vi "Sub Super Duper_14_02_18_JWa.vi"(0 "VISA resource name":refnum<visa-resource-name>="GPIB0::17::INSTR", 1 "Sample Properties:":T9 {"Date Created" format="%<%Y/%m/%d>T"}, 2 "Gated SMU4 is...":bool, 3 "TRF Cluster":T10={"Step 4"=-38.0, "# of Loops"=1.0, "Transfer 2"=FALSE, "Start 4"=-2.0, "Total Points 2"=2, "Start 3"=40.0, "Stop 2"=-40.0, "Step 3"=-1.0, "Loop Step"=0.0, "Integration Time 3"=0, "Loop Wait"=0.0, "First Step"=0.0} {"Loop Wait" format="%<%H:%M:%S>t"; "Integration Time 3" scale=0.0..2.0; "Step 3" format="%.2f"; "Stop 2" format="%.2f"; "Start 3" format="%.2f"; "Start 4" format="%.2f"; "Step 4" format="%.2f"}, 4 "TSP Cluster":T11={"Transport"=FALSE, "Start 2"=0.0, "Stop 3"=-60.0, "Step 2"=-1.0, "Start"=0.0, "Step"=-10.0, "Total Points"=7, "Integration Time"=0} {"Integration Time" scale=0.0..2.0; "Step" format="%.2f"; "Start" format="%.2f"; "Step 2" format="%.2f"; "Stop 3" format="%.2f"; "Start 2" format="%.2f"}, 5 "Compliance Cluster":T6={"Var1 sweep settings"={"sweep spacing (linear: 0)"=0, "sweep mode"=FALSE, "compliance (V)"=100.0, "compliance (A)"=0.001}, "Var1 sweep settings 2"={"sweep spacing (linear: 0)"=0, "sweep mode"=FALSE, "compliance (V)"=100.0, "compliance (A)"=0.001}, "Var2 step settings 2"={"compliance (A)"=0.001, "compliance (V)"=100.0}, "Var2 step settings"={"compliance (A)"=0.001, "compliance (V)"=100.0}} {"Var2 step settings"."compliance (V)" format="%.2f"; "Var2 step settings"."compliance (A)" format="%^.2e"; "Var2 step settings 2"."compliance (V)" format="%.2f"; "Var2 step settings 2"."compliance (A)" format="%^.2e"; "Var1 sweep settings 2"."compliance (A)" format="%^.2e"; "Var1 sweep settings 2"."compliance (V)" format="%.2f"; "Var1 sweep settings 2"."sweep spacing (linear: 0)" items=["linear", "log 10", "log 25", "log 50"]; "Var1 sweep settings"."compliance (A)" format="%^.2e"; "Var1 sweep settings"."compliance (V)" format="%.2f"; "Var1 sweep settings"."sweep spacing (linear: 0)" items=["linear", "log 10", "log 25", "log 50"]}, 6 "Light Bathe Cluster":T2={"TG to BG:  "=FALSE, "TG to BG Durration"=120.0, "TRF to TSP:   "=FALSE, "TRF to TSP Duration"=120.0, "Post Measure: "=FALSE, "TG to BG (TSP):"=FALSE, "TG to BG Durration 3"=120.0} {"TG to BG Durration 3" format="%<%H:%M:%S>t"; "TRF to TSP Duration" format="%<%H:%M:%S>t"; "TG to BG Durration" format="%<%H:%M:%S>t"}, 7 "error in":errorcluster, 8 "Saved Folder:":path=path "C:/1DATA/2011", 9 "Wait Cluster":T5 {"Wait Time (s)" format="%.1g"; "Wait Countdown" format="%<%H:%M:%S%1u>t"}, 11 "TG Dielectric Prop":T1, 13 "Stop \nCountdown":bool, 15 "Loop Count":dbl, 16 "Gate Current Cluster":T3={"Gate Current (TSP)"={"Y2 axis on/off"=FALSE, "MINIMUM"=0.0, "MAXIMUM"=1.0, "Variable name"="Ig", "LIN or LOG axis"="LIN"}, "Gate Current (TRF)"={"Y2 axis on/off"=FALSE, "MINIMUM"=0.0, "MAXIMUM"=1.0, "Variable name"="Ig", "LIN or LOG axis"="LIN"}} {"Gate Current (TSP)"."MAXIMUM" format="%.9f"; "Gate Current (TSP)"."MINIMUM" format="%.9f"; "Gate Current (TRF)"."MAXIMUM" format="%.9f"; "Gate Current (TRF)"."MINIMUM" format="%.9f"}, 17 "Dielectric Constant (BG)":dbl) -> (12 "Status Indicator":bool, 14 "Vt Cluster":T4 {"Id Max" format="%.3g"; "Vt Max" format="%.3g"; "Vt Min" format="%.3g"; "Vt Ratio" format="%.3g"}, 20 "VISA resource name out":refnum<visa-resource-name>, 21 "TRF Path":path, 23 "TSP Path":path, 24 "Graph Cluster":T7, 25 "Char Cluster":T8 {"Mobility-Lin" format="%#_4e"; "On/Off" format="%#_4e"; "Mobility-Sat" format="%#_4e"}, 27 "error out":errorcluster)   [LabVIEW 2012]
uses:
  <vilib>/Platform/TimedLoop/XDataNode/wakeup.ctl
  <vilib>/Platform/TimedLoop/XDataNode/XDNodeRunTimeDep.lvlib
  <vilib>/Platform/TimedLoop/XDataNode/nitl_modes.ctl
  <vilib>/Platform/TimedLoop/XDataNode/timing_clust.ctl
  <vilib>/Platform/TimedLoop/XDataNode/XDataNode.xnode
panel:
  out "LKG Path":path
  # "Vg Sweep"
  # "Vd Step"
  # "Loops and Integration Time"
  # "Device Characteristics"
  # "Light Bath is..."
  # "Duration (hh:mm:ss)"
  # "Sample Properties:"
  # "%"
  # "nm"
  # "Device Properties:"
  # "um"
  # "um"
  # "Vg Step"
  # "Vd Step"
  # "Integration Time"
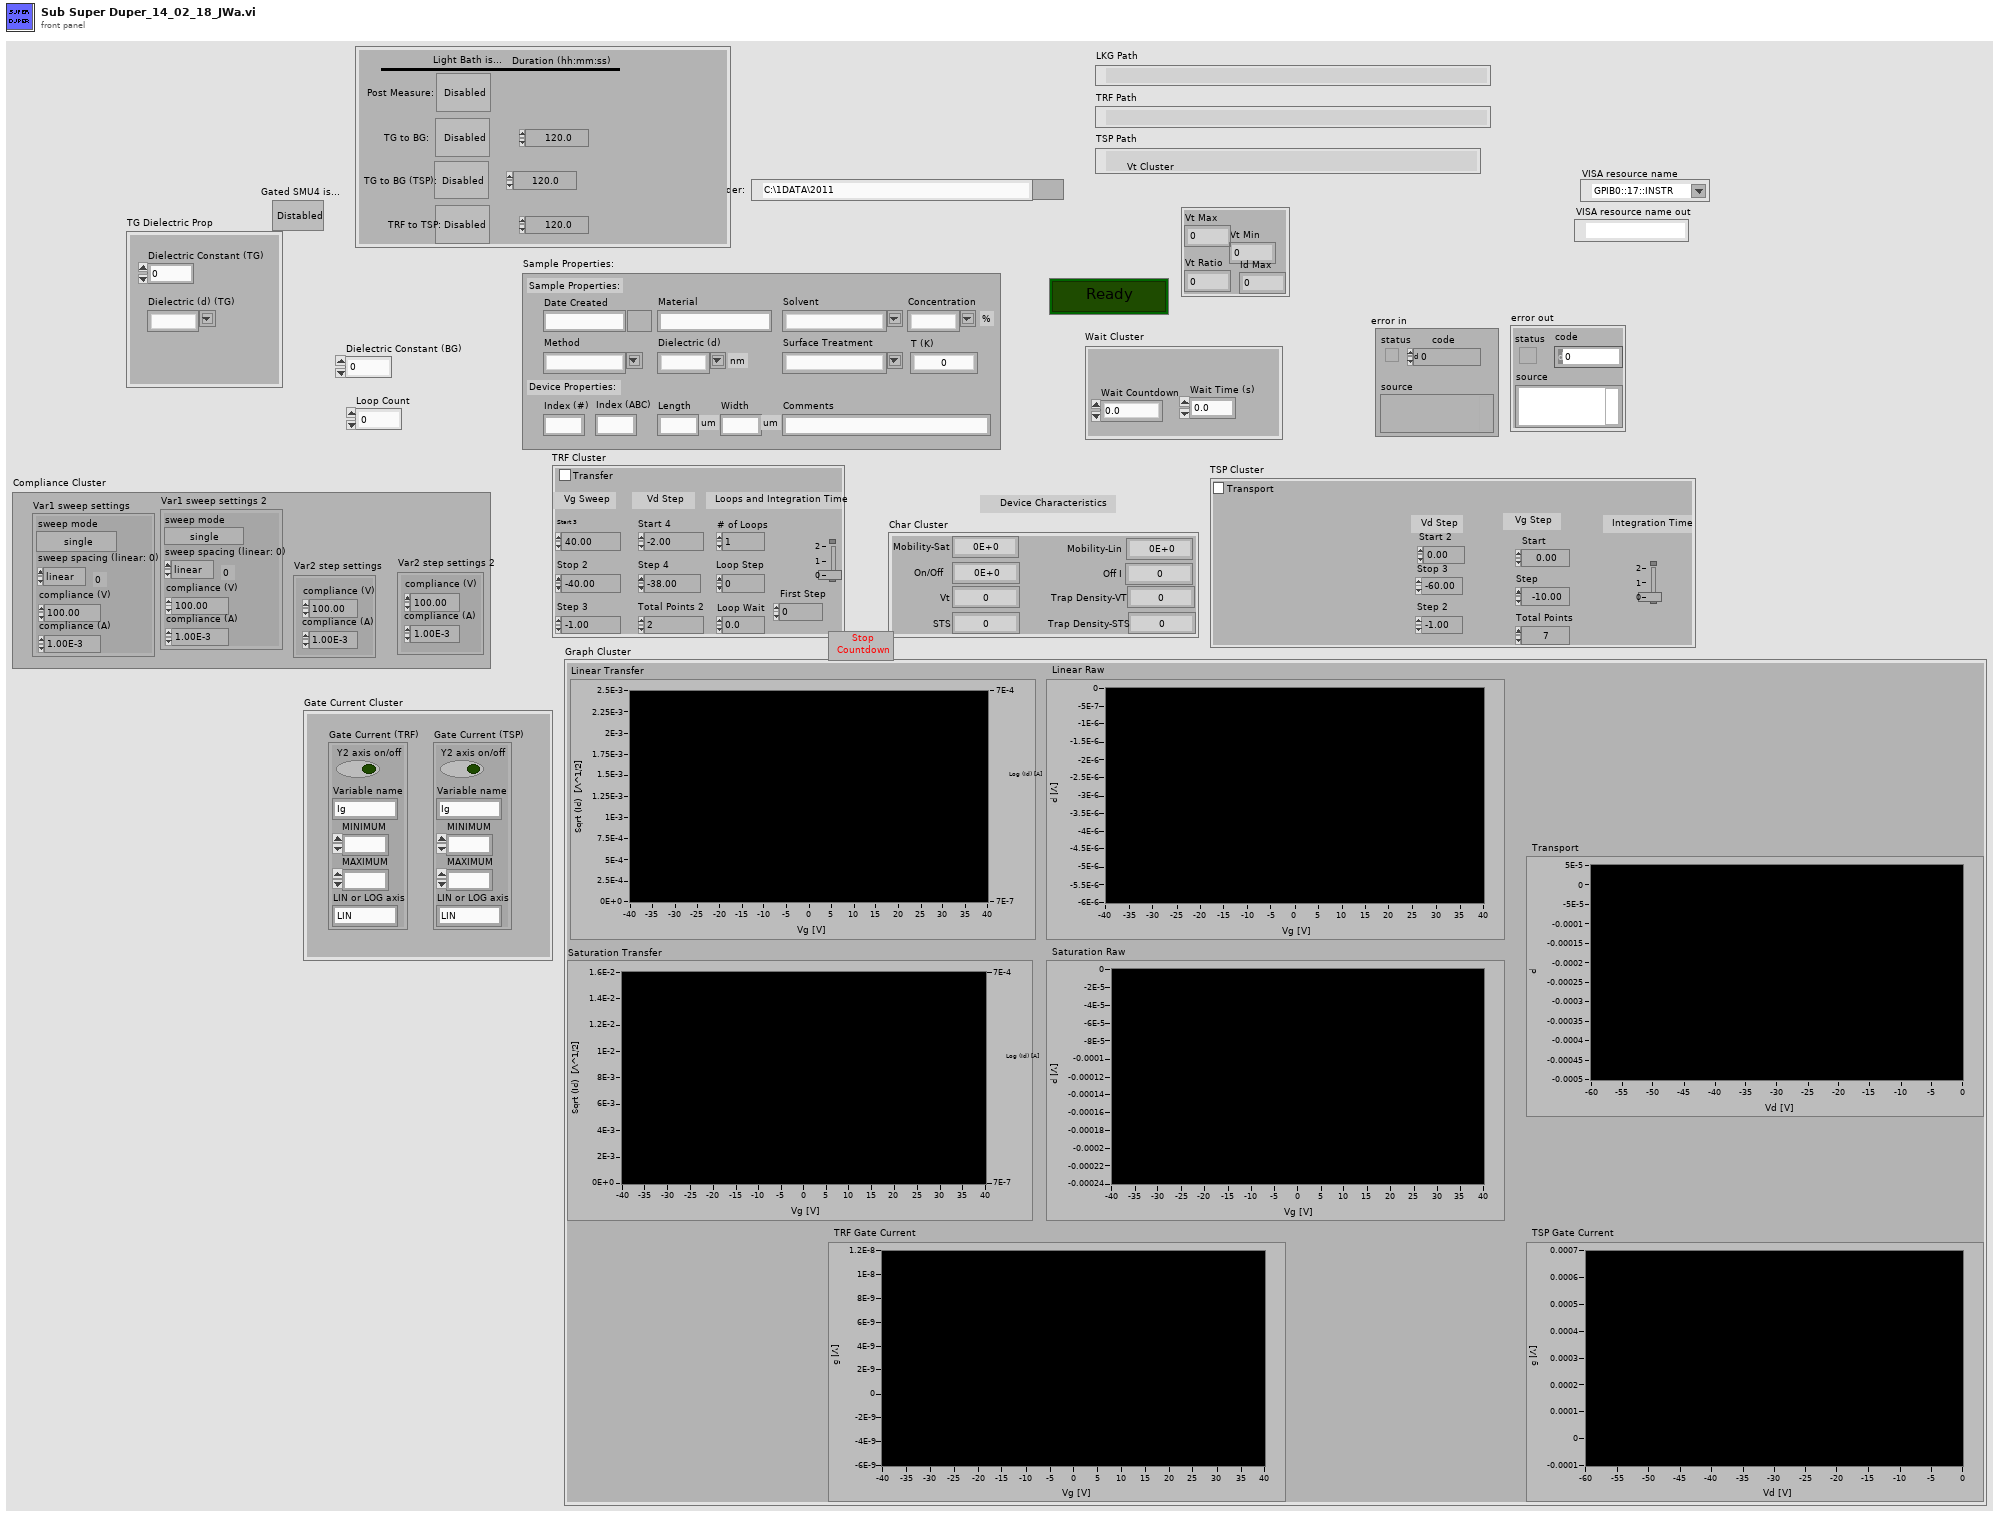
[diagram p1: front panel]
types:
  T1 = cluster{"Dielectric Constant (TG)":dbl, "Dielectric (d) (TG)":string}
  T2 = cluster{"TG to BG:  ":bool, "TG to BG Durration":dbl, "TRF to TSP:   ":bool, "TRF to TSP Duration":dbl, "Post Measure: ":bool, "TG to BG (TSP):":bool, "TG to BG Durration 3":dbl}
  T3 = cluster{"Gate Current (TSP)":cluster{"Y2 axis on/off":bool, "MINIMUM":ext, "MAXIMUM":ext, "Variable name":string, "LIN or LOG axis":string}, "Gate Current (TRF)":cluster{"Y2 axis on/off":bool, "MINIMUM":ext, "MAXIMUM":ext, "Variable name":string, "LIN or LOG axis":string}}
  T4 = cluster{"Vt Max":i32, "Vt Min":i32, "Vt Ratio":i32, "Id Max":i32}
  T5 = cluster{"Wait Countdown":dbl, "Wait Time (s)":dbl}
  T6 = cluster{"Var1 sweep settings":cluster{"sweep spacing (linear: 0)":u16, "sweep mode":bool, "compliance (V)":dbl, "compliance (A)":dbl}, "Var1 sweep settings 2":cluster{"sweep spacing (linear: 0)":u16, "sweep mode":bool, "compliance (V)":dbl, "compliance (A)":dbl}, "Var2 step settings 2":cluster{"compliance (A)":dbl, "compliance (V)":dbl}, "Var2 step settings":cluster{"compliance (A)":dbl, "compliance (V)":dbl}}
  T7 = cluster{"Linear Transfer":cluster{dbl[], "trace":dbl[]}[], "Linear Raw":cluster{dbl[], dbl[]}[], "Saturation Transfer":cluster{dbl[], "trace":dbl[]}[], "Saturation Raw":cluster{dbl[], dbl[]}[], "Transport":cluster{dbl[], dbl[]}[], "TRF Gate Current":cluster{dbl[], dbl[]}[], "TSP Gate Current":cluster{dbl[], dbl[]}[]}
  T8 = cluster{"Mobility-Sat":dbl, "Mobility-Lin":dbl, "On/Off ":dbl, "Off I":dbl, "Vt":dbl, "STS":dbl, "Trap Density-VT":dbl, "Trap Density-STS":dbl}
  T9 = cluster{"Date Created":timestamp, "Material":string, "Solvent":string, "Concentration":string, "Method":string, "Dielectric (d)":string, "Index (#)":string, "Index (ABC)":string, "Length":string, "Width":string, "Surface Treatment":string, "Comments":string, "T (K)":dbl}
  T10 = cluster{"Step 4":dbl, "# of Loops":dbl, "Transfer 2":bool, "Start 4":dbl, "Total Points 2":u16, "Start 3":dbl, "Stop 2":dbl, "Step 3":dbl, "Loop Step":dbl, "Integration Time 3":u32, "Loop Wait":dbl, "First Step":dbl}
  T11 = cluster{"Transport":bool, "Start 2":dbl, "Stop 3":dbl, "Step 2":dbl, "Start":dbl, "Step":dbl, "Total Points":u16, "Integration Time":u32}
  T12 = typedef "XDNodeRunTimeDep.lvlib/timing_clust.ctl" = cluster{"Expected End [f-1]":u64, "Actual End [f-1]":u64, "Finished Late? [f-1]":bool, "Expected End [i-1]":u64, "Actual End [i-1]":u64, "Finished Late? [i-1]":bool, "Expected Start [i]":u64, "Actual Start [i]":u64, "Expected Start [f]":u64, "Actual Start [f]":u64, "Source Name":string, "Structure Name":string, "Period":i64, "Deadline":i64, "Offset":i64, "Start":i64, "Priority":i32, "Timeout":i32, "Mode":T13, "Wakeup Reason":T14, "Error":errorcluster, "Source Type":string, "Secondary Source Type":string, "Global End Time":u64, "Global Start Time":u64, "Frame Duration":u64, "Iteration Duration":u64, "Assigned CPU":i32, "I/O Scan Engine Mode":u32}
  T13 = typedef "XDNodeRunTimeDep.lvlib/nitl_modes.ctl" = enum32{"No Change", "Process missed periods, maintain original phase", "Discard missed periods, maintain original phase", "Process missed periods, ignore original phase", "Discard missed periods, ignore original phase"}
  T14 = typedef "XDNodeRunTimeDep.lvlib/wakeup.ctl" = enum32{"Normal", "Aborted", "Asynchronous wakeup", "Timing source error", "Timed loop error", "Timeout"}
  T15 = cluster{"sweep spacing (linear: 0)":u16, "sweep mode":bool, "compliance (V)":dbl, "compliance (A)":dbl}
  T16 = cluster{"compliance (A)":dbl, "compliance (V)":dbl}
  T17 = cluster{"Y2 axis on/off":bool, "MINIMUM":ext, "MAXIMUM":ext, "Variable name":string, "LIN or LOG axis":string}
  T18 = cluster{"Start 3":dbl, "Stop 2":dbl, "Step 3":dbl, "sweep spacing (linear: 0)":u16, "sweep mode":bool, "compliance (V)":dbl, "compliance (A)":dbl}
  T19 = cluster{"compliance (A)":dbl, "compliance (V)":dbl, "Start 4":dbl, "Total Points 2":u16, dbl}
  T20 = cluster{"Vt Max":i32, "Vt Min":i32, "Vt Ratio":i32, "Id Max":dbl}
  T21 = cluster{"Mobility-Sat":dbl, "Mobility-Lin":dbl, "On/Off Current":dbl, "Off I":dbl, "Vt":dbl, "STS":dbl, "Trap Density-VT":dbl, "Trap Density-STS":dbl}
  T22 = cluster{"Linear Sqrt":cluster{dbl[], "trace":dbl[]}[], "Linear Log":cluster{dbl[], "trace":dbl[]}[], "Linear Raw":cluster{dbl[], dbl[]}[], "Saturation Sqrt":cluster{dbl[], "trace":dbl[]}[], "Saturation Log":cluster{dbl[], "trace":dbl[]}[], "Saturation Raw":cluster{dbl[], "trace":dbl[]}[], "Gate Current":cluster{dbl[], "trace":dbl[]}[]}
  T23 = cluster{"Start 2":dbl, "Stop 3":dbl, "Step 2":dbl, "sweep spacing (linear: 0)":u16, "sweep mode":bool, "compliance (V)":dbl, "compliance (A)":dbl}
  T24 = cluster{"compliance (A)":dbl, "compliance (V)":dbl, "Start":dbl, "Total Points":u16, "Step":dbl}
  T25 = cluster{"Transport":cluster{dbl[], dbl[]}[], "Gate Current":cluster{dbl[], dbl[]}[]}
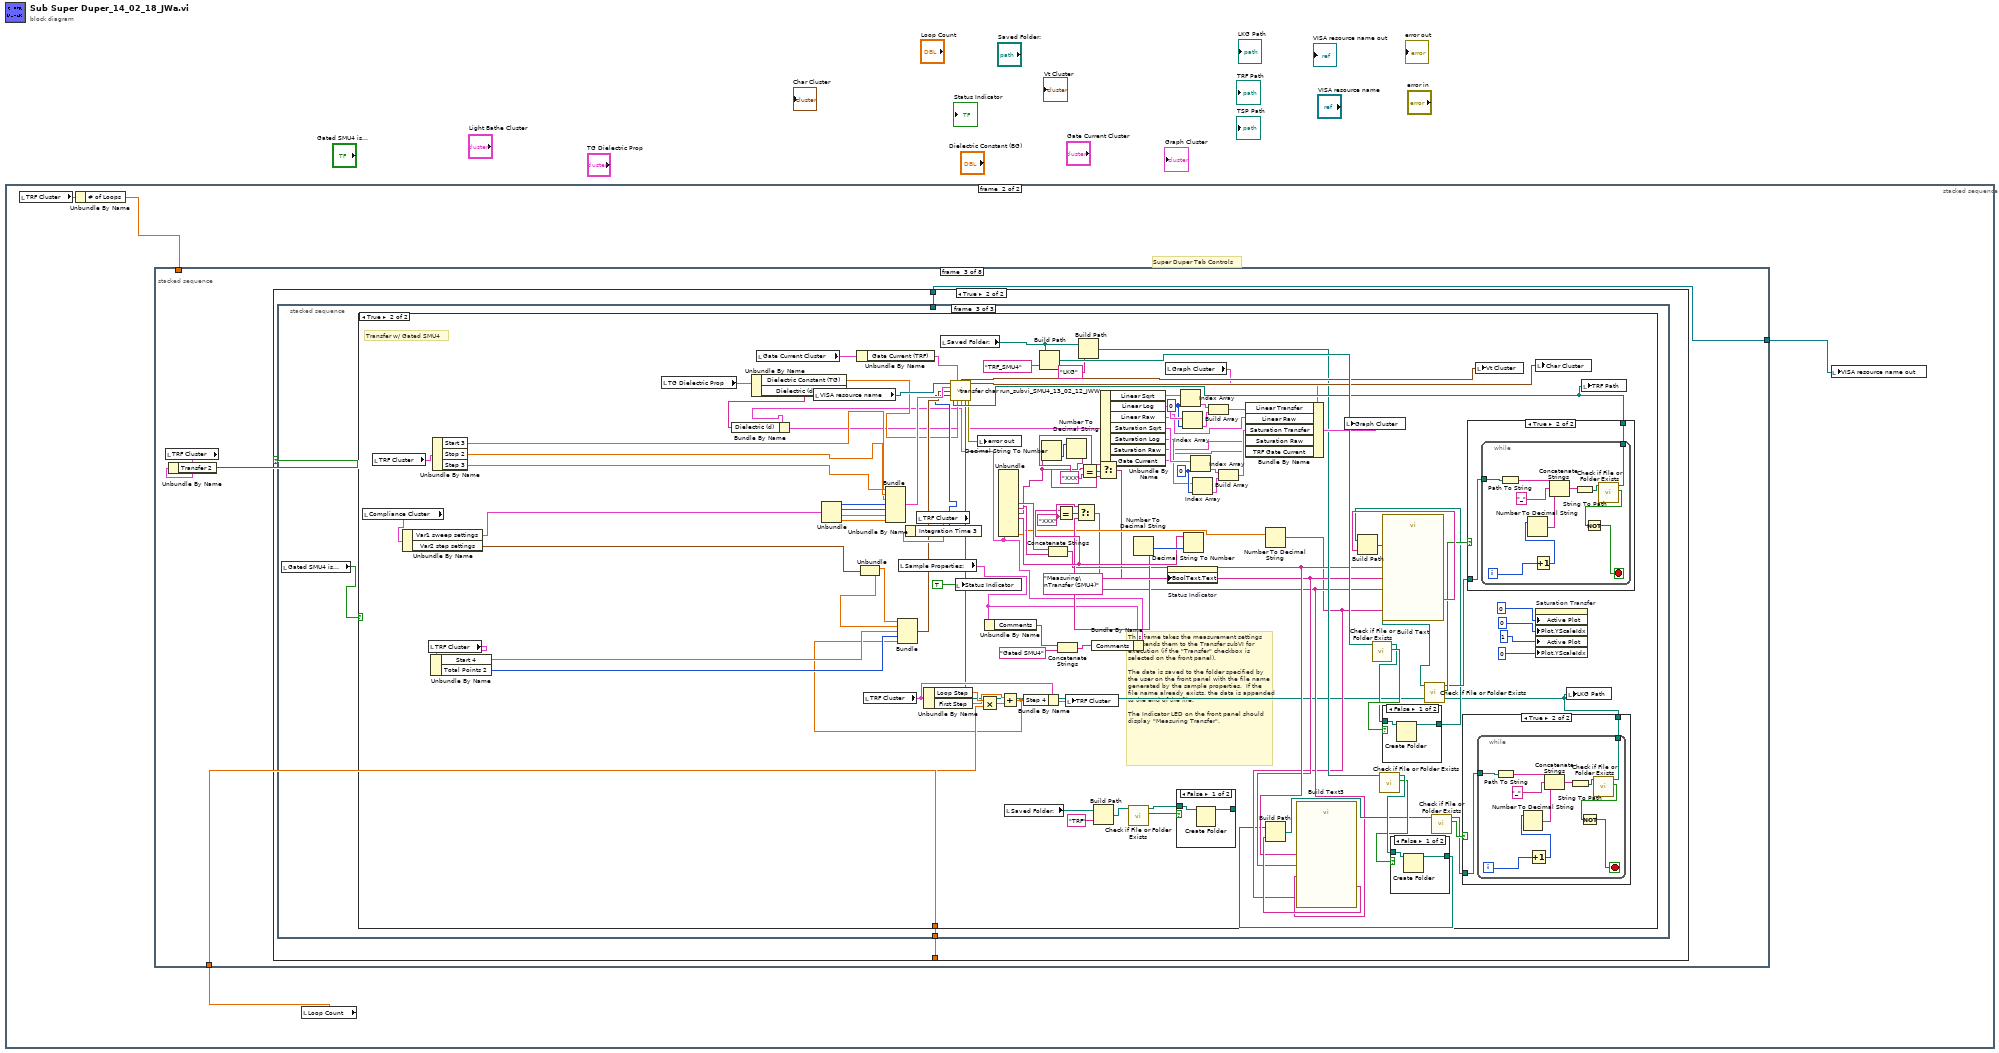
[diagram p0: block diagram]
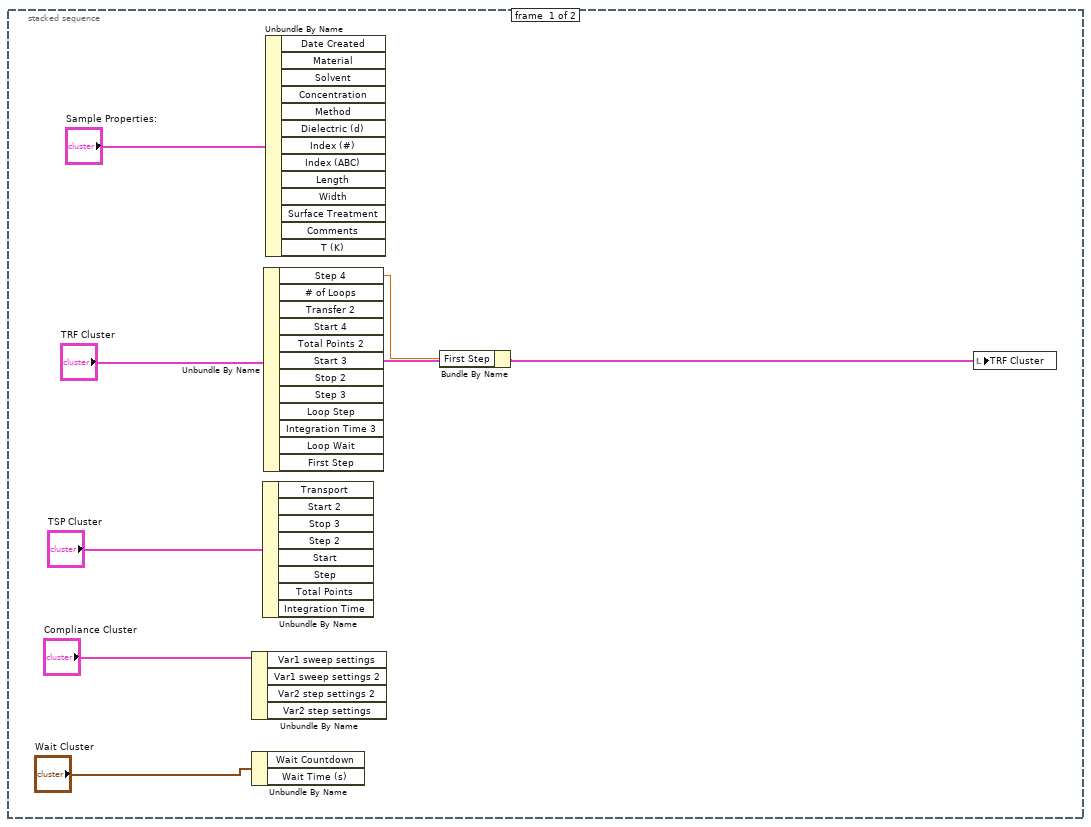
[diagram p2: hidden frame]
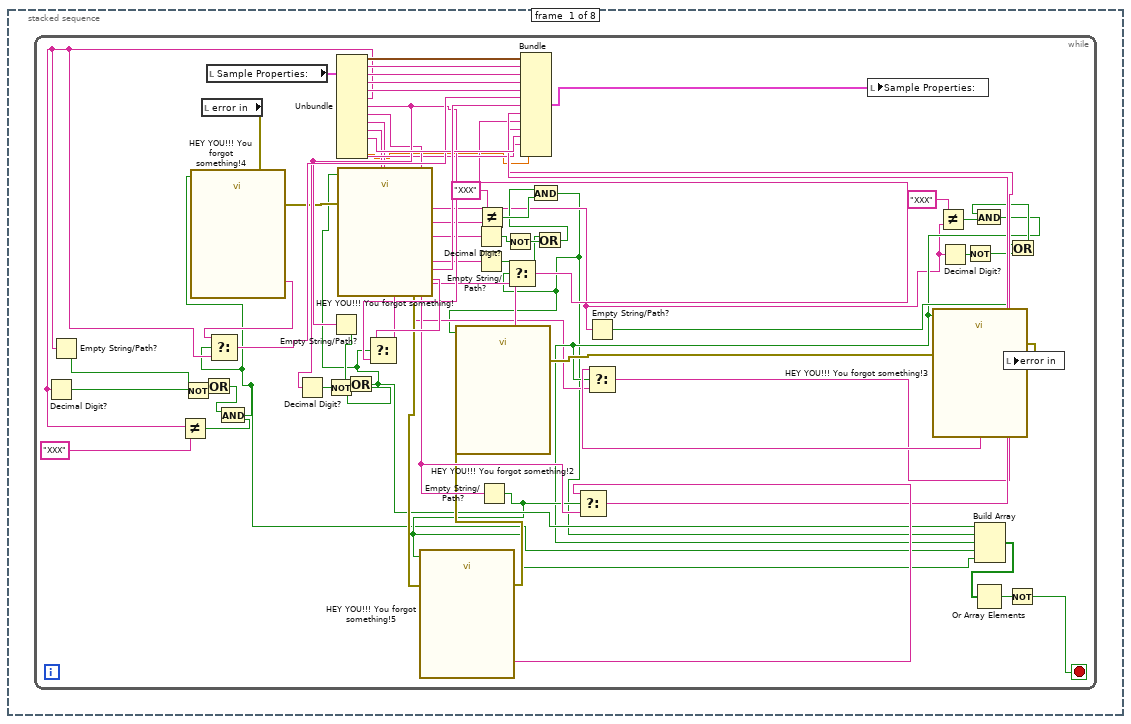
[diagram p3: hidden frame]
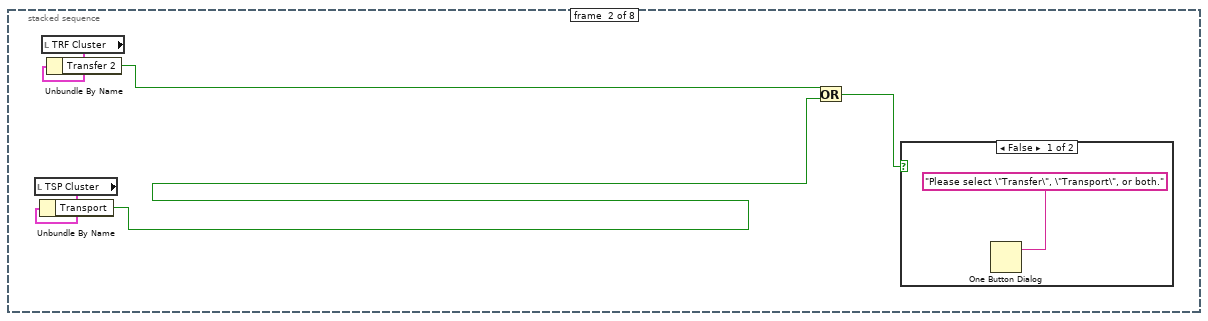
[diagram p4: hidden frame]
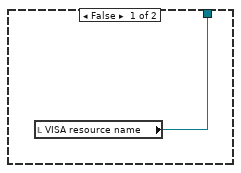
[diagram p6: hidden frame]
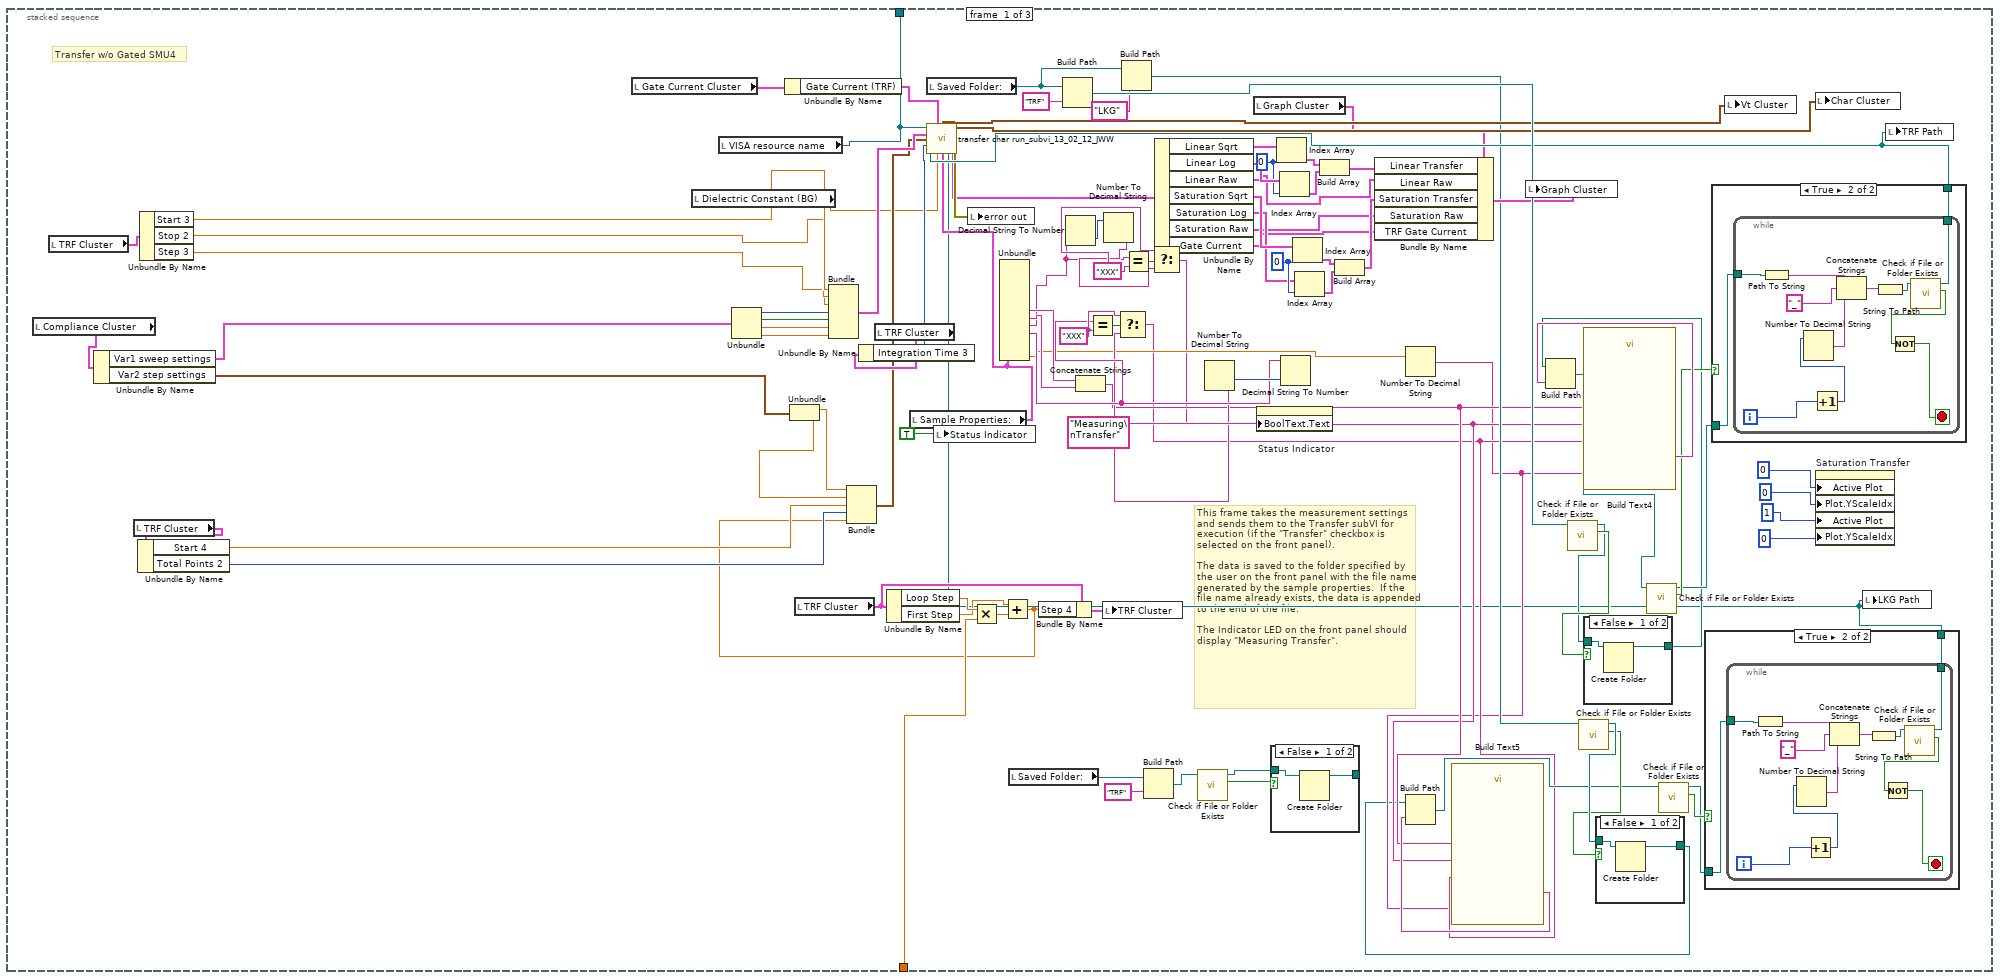
[diagram p7: hidden frame]
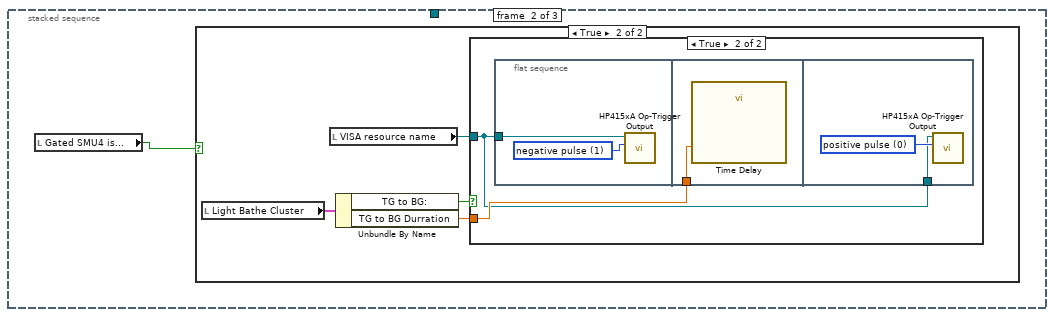
[diagram p13: hidden frame]
diagram:
  n1 = stacked-sequence {
    frame #0 {
      n2 = Unbundle By Name("Compliance Cluster") -> ()  [unwired: 4 out]
      n3 = Unbundle By Name("Wait Cluster") -> ()  [unwired: 2 out]
      n4 = Unbundle By Name("TSP Cluster") -> ()  [unwired: 8 out]
      n5 = Unbundle By Name("TRF Cluster") -> ("Step 4"=w7:dbl)  [unwired: 11 out]
      n6 = Unbundle By Name("Sample Properties:") -> ()  [unwired: 13 out]
      n7 = Bundle By Name(cluster="TRF Cluster", "First Step"=w7) -> (w5:T10)
      n8 = local write "TRF Cluster"(w5) -> ()
    }
    frame #1 {
      # "Super Duper Tab Controls"
      n9 = local read "TRF Cluster"() -> (w11:T10)
      n10 = Unbundle By Name(w11) -> ("# of Loops"=w10:dbl)
      n11 = local read "Loop Count"() -> (w8:dbl)
      n12 = stacked-sequence {
        tunnel: w8 -> [_ _ w81 _ _ _ _ w596]
        tunnel: w10 -> [_ _ _ _ _ _ _ w595]
        tunnel: [_ _ w78 _ _ _ _ _] -> w9
        frame #0 {
          n13 = while {
            stop <- w37 stop-if-true
            n14 = local read "error in"() -> (w43:errorcluster)
            n15 = local read "Sample Properties:"() -> (w66:T9)
            n16 = Unbundle(w66) -> ("Date Created"=w67:timestamp, "Material"=w68:string, "Solvent"=w69:string, "Concentration"=w70:string, "Method"=w71:string, "Dielectric (d)"=w26:string, "Index (#)"=w56:string, "Index (ABC)"=w53:string, "Length"=w21:string, "Width"=w14:string, "Surface Treatment"=w59:string, "Comments"=w51:string, "T (K)"=w12:dbl)
            n17 = Decimal Digit?(1:w26) -> (0:w34:bool)
            n18 = Empty String/Path?(string/path=w26) -> (empty?=w28:bool)
            n19 = Not Equal?(x=w26, y="XXX") -> (x != y?=w25:bool)
            n20 = Not(x=w34) -> (.not. x?=w31:bool)
            n21 = Or(x=w28, y=w31) -> (x .or. y?=w24:bool)
            n22 = And(x=w24, y=w25) -> (x .and. y?=w23:bool)
            n23 = call "HEY YOU!!! You forgot something!4"("Enable"=w23, "error in (no error)"=w43) -> ("Dielectric (d)"=w58:string, "error out"=w42:errorcluster)  [unwired: 15 in, 1 out]
            n24 = Select(t=w58, s=w23, f=w26) -> (s? t:f=w57:string)
            n25 = Decimal Digit?(1:w56) -> (0:w47:bool)
            n26 = Not(x=w47) -> (.not. x?=w46:bool)
            n27 = Empty String/Path?(string/path=w56) -> (empty?=w55:bool)
            n28 = Or(x=w55, y=w46) -> (x .or. y?=w41:bool)
            n29 = call "HEY YOU!!! You forgot something!"("Enable"=w41, "error in (no error)"=w42) -> ("Index (#)"=w65:string, "error out"=w45:errorcluster)  [unwired: 15 in, 1 out]
            n30 = Select(t=w65, s=w41, f=w56) -> (s? t:f=w62:string)
            n31 = Decimal Digit?(1:w21) -> (0:w36:bool)
            n32 = Empty String/Path?(string/path=w21) -> (empty?=w30:bool)
            n33 = Not Equal?(x="XXX", y=w21) -> (x != y?=w20:bool)
            n34 = Empty String/Path?(string/path=w53) -> (empty?=w40:bool)
            n35 = call "HEY YOU!!! You forgot something!5"("Enable"=w40, "error in (no error)"=w45) -> ("Index (ABC)"=w54:string, "error out"=w44:errorcluster)  [unwired: 15 in, 1 out]
            n36 = Not(x=w36) -> (.not. x?=w33:bool)
            n37 = Or(x=w30, y=w33) -> (x .or. y?=w19:bool)
            n38 = And(x=w19, y=w20) -> (x .and. y?=w13:bool)
            n39 = call "HEY YOU!!! You forgot something!2"("Enable"=w13, "error in (no error)"=w44) -> ("Length"=w64:string, "error out"=w61:errorcluster)  [unwired: 15 in, 1 out]
            n40 = Select(t=w64, s=w13, f=w21) -> (s? t:f=w50:string)
            n41 = Select(t=w54, s=w40, f=w53) -> (s? t:f=w52:string)
            n42 = Empty String/Path?(string/path=w14) -> (empty?=w29:bool)
            n43 = Not Equal?(x="XXX", y=w14) -> (x != y?=w18:bool)
            n44 = Decimal Digit?(1:w14) -> (0:w35:bool)
            n45 = Not(x=w35) -> (.not. x?=w32:bool)
            n46 = Or(x=w29, y=w32) -> (x .or. y?=w17:bool)
            n47 = And(x=w17, y=w18) -> (x .and. y?=w16:bool)
            n48 = call "HEY YOU!!! You forgot something!3"("Enable"=w16, "error in (no error)"=w61) -> ("Width"=w63:string, "error out"=w60:errorcluster)  [unwired: 15 in, 1 out]
            n49 = Select(t=w63, s=w16, f=w14) -> (s? t:f=w49:string)
            n50 = Bundle("Date Created"=w67, "Material"=w68, "Solvent"=w69, "Concentration"=w70, "Method"=w71, "Dielectric (d)"=w57, "Index (#)"=w62, "Index (ABC)"=w52, "Length"=w50, "Width"=w49, "Surface Treatment"=w59, "Comments"=w51, "T (K)"=w12) -> (w48:T9)  [unwired: 1 in]
            n51 = local write "Sample Properties:"(w48) -> ()
            n52 = Build Array(w41, w13, w16, w23, w40) -> (w39:bool[])
            n53 = Or Array Elements(Boolean array=w39) -> (logical OR=w38:bool)
            n54 = local write "error in"(w60) -> ()
            n55 = Not(x=w38) -> (.not. x?=w37:bool)
          }
        }
        frame #1 {
          n56 = local read "TSP Cluster"() -> (w73:T11)
          n57 = Unbundle By Name(w73) -> ("Transport"=w72:bool)
          n58 = local read "TRF Cluster"() -> (w75:T10)
          n59 = Unbundle By Name(w75) -> ("Transfer 2"=w74:bool)
          n60 = Or(x=w74, y=w72) -> (x .or. y?=w76:bool)
          n61 = case shown="False" w76 {
            frame False {
              n62 = One Button Dialog(message="Please select \"Transfer\", \"Transport\", or both.") -> ()  [unwired: 1 in, 1 out]
            }
            frame True {
            }
          }
        }
        frame #2 {
          n63 = local read "TRF Cluster"() -> (w79:T10)
          n64 = Unbundle By Name(w79) -> ("Transfer 2"=w80:bool)
          n65 = case shown="True" w80 {
            tunnel: w81 -> [_ w84]
            tunnel: [w82 w83] -> w78
            frame False {
              n66 = local read "VISA resource name"() -> (w82:refnum<visa-resource-name>)
            }
            frame True {
              n67 = stacked-sequence {
                tunnel: w84 -> [w186 _ w237]
                tunnel: [w185 _ _] -> w83
                frame #0 {
                  w115 = 0
                  w121 = 0
                  w164 = "XXX"
                  w167 = "XXX"
                  # "Transfer w/o Gated SMU4"
                  # "This frame takes the measurement settings and sends them to the Transfer subVI for execution (if the \"Transfer\" checkbox is selected on the front panel).\n\nThe data is saved to the folder specified by the user on the front panel with the file name generated by the sample properties.  If the file name already exists, the data is appended to the end of the file.\n\nThe Indicator LED on the front panel should display \"Measuring Transfer\"."
                  n68 = local read "Compliance Cluster"() -> (w143:T6)
                  n69 = local read "TRF Cluster"() -> (w148:T10)
                  n70 = Unbundle By Name(w143) -> ("Var1 sweep settings"=w141:T15, "Var2 step settings"=w142:T16)
                  n71 = local read "TRF Cluster"() -> (w151:T10)
                  n72 = Unbundle By Name(w151) -> ("Start 4"=w150:dbl, "Total Points 2"=w149:u16)
                  n73 = Unbundle By Name(w148) -> ("Start 3"=w147:dbl, "Stop 2"=w146:dbl, "Step 3"=w145:dbl)
                  n74 = local read "Gate Current Cluster"() -> (w87:T3)
                  n75 = local read "Dielectric Constant (BG)"() -> (w85:dbl)
                  n76 = local read "VISA resource name"() -> (w185:refnum<visa-resource-name>)
                  n77 = Unbundle(w141) -> ("sweep spacing (linear: 0)"=w184:u16, "sweep mode"=w183:bool, "compliance (V)"=w182:dbl, "compliance (A)"=w181:dbl)
                  n78 = Unbundle By Name(w87) -> ("Gate Current (TRF)"=w86:T17)
                  n79 = Unbundle(w142) -> ("compliance (A)"=w180:dbl, "compliance (V)"=w179:dbl)
                  n80 = local read "TRF Cluster"() -> (w134:T10)
                  n81 = Bundle("Start 3"=w147, "Stop 2"=w146, "Step 3"=w145, "sweep spacing (linear: 0)"=w184, "sweep mode"=w183, "compliance (V)"=w182, "compliance (A)"=w181) -> (w133:T18)  [unwired: 1 in]
                  n82 = local read "TRF Cluster"() -> (w144:T10)
                  n83 = Unbundle By Name(w144) -> ("Integration Time 3"=w131:u32)
                  n84 = Unbundle By Name(w134) -> ("Loop Step"=w137:dbl, "First Step"=w136:dbl)
                  n85 = local read "Sample Properties:"() -> (w129:T9)
                  n86 = local read "Saved Folder:"() -> (w102:path)
                  n87 = local write "Status Indicator"(TRUE) -> ()
                  n88 = Multiply(x=w137, y=w186) -> (x*y=w139:dbl)
                  n89 = Unbundle(w129) -> ("Index (#)"=w175:string, "Index (ABC)"=w174:string, "Length"=w161:string, "Width"=w163:string, "T (K)"=w140:dbl)  [unwired: 8 out]
                  n90 = Add(x=w136, y=w139) -> (x+y=w135:dbl)
                  n91 = Bundle("compliance (A)"=w180, "compliance (V)"=w179, "Start 4"=w150, "Total Points 2"=w149, w135) -> (w132:T19)  [unwired: 1 in]
                  n92 = local read "Saved Folder:"() -> (w108:path)
                  n93 = Bundle By Name(cluster=w134, "Step 4"=w135) -> (w138:T10)
                  n94 = Build Path(base path=w102, name or relative path="TRF") -> (appended path=w157:path)
                  n95 = Decimal String To Number(string=w161) -> (number=w170:i32)  [unwired: 2 in, 1 out]
                  n96 = Concatenate Strings(w175, w174) -> (w93:string)
                  n97 = Equal?(x=w163, y=w164) -> (x = y?=w165:bool)
                  n98 = local write "TRF Cluster"(w138) -> ()
                  n99 = Number To Decimal String(number=w170) -> (decimal integer string=w166:string)  [unwired: 1 in]
                  n100 = Build Path(base path=w102, name or relative path="LKG") -> (appended path=w98:path)
                  n101 = Equal?(x=w161, y=w167) -> (x = y?=w168:bool)
                  n102 = Build Path(base path=w108, name or relative path="TRF") -> (appended path=w106:path)
                  n103 = Select(t=w167, s=w168, f=w166) -> (s? t:f=w92:string)
                  n104 = call <vilib>:"Check if File or Folder Exists.vi"("path"=w106) -> ("file or folder exists?"=w104:bool, "dup path"=w105:path)  [unwired: 8 in, 1 out]
                  n105 = local read "Graph Cluster"() -> (w124:T7)
                  n106 = property on="Status Indicator" class="Bool (strict)"("BoolText.Text"="Measuring\nTransfer") -> ()  [unwired: 2 in, 2 out]
                  n107 = case shown="False" w104 {
                    tunnel: w105 -> [w205 w206]
                    tunnel: [w204 w206] -> _
                    frame False {
                      n108 = Create Folder(path (use dialog)=w205) -> (created path=w204:path)  [unwired: 2 in, 2 out]
                    }
                    frame True {
                    }
                  }
                  n109 = Decimal String To Number(string=w163) -> (number=w169:i32)  [unwired: 2 in, 1 out]
                  n110 = Number To Decimal String(number=w169) -> (decimal integer string=w162:string)  [unwired: 1 in]
                  n111 = Select(t=w164, s=w165, f=w162) -> (s? t:f=w91:string)
                  n112 = Number To Decimal String(number=w140) -> (decimal integer string=w90:string)  [unwired: 1 in]
                  n113 = call "Build Text5"("T"=w90, "Index"=w93, "Length"=w92, "Width"=w91) -> ("Result"=w94:string)  [unwired: 10 in, 1 out]
                  n114 = call <vilib>:"Check if File or Folder Exists.vi"("path"=w157) -> ("file or folder exists?"=w159:bool, "dup path"=w158:path)  [unwired: 8 in, 1 out]
                  n115 = call <vilib>:"Check if File or Folder Exists.vi"("path"=w98) -> ("file or folder exists?"=w99:bool, "dup path"=w100:path)  [unwired: 8 in, 1 out]
                  n116 = call "Build Text4"("T"=w90, "Index"=w93, "Length"=w92, "Width"=w91) -> ("Result"=w178:string)  [unwired: 10 in, 1 out]
                  n117 = case shown="False" w159 {
                    tunnel: w158 -> [w208 w209]
                    tunnel: [w207 w209] -> w156
                    frame False {
                      n118 = Create Folder(path (use dialog)=w208) -> (created path=w207:path)  [unwired: 2 in, 2 out]
                    }
                    frame True {
                    }
                  }
                  n119 = Build Path(base path=w156, name or relative path=w178) -> (appended path=w172:path)
                  n120 = case shown="False" w99 {
                    tunnel: w100 -> [w202 w203]
                    tunnel: [w201 w203] -> w89
                    frame False {
                      n121 = Create Folder(path (use dialog)=w202) -> (created path=w201:path)  [unwired: 2 in, 2 out]
                    }
                    frame True {
                    }
                  }
                  n122 = Build Path(base path=w89, name or relative path=w94) -> (appended path=w97:path)
                  n123 = call <vilib>:"Check if File or Folder Exists.vi"("path"=w172) -> ("file or folder exists?"=w173:bool, "dup path"=w171:path)  [unwired: 8 in, 1 out]
                  n124 = call <vilib>:"Check if File or Folder Exists.vi"("path"=w97) -> ("file or folder exists?"=w96:bool, "dup path"=w95:path)  [unwired: 8 in, 1 out]
                  n125 = case shown="True" w96 {
                    tunnel: w95 -> [w187 w189]
                    tunnel: [w187 w188] -> w88
                    frame False {
                    }
                    frame True {
                      n126 = while {
                        tunnel: w189 -> [w191]
                        tunnel: [w190] -> w188
                        i -> [w193]
                        stop <- w194 stop-if-true
                        n127 = Path To String(path=w191) -> (string=w200:string)
                        n128 = Increment(x=w193) -> (x+1=w192:i32)
                        n129 = Number To Decimal String(number=w192) -> (decimal integer string=w198:string)  [unwired: 1 in]
                        n130 = Concatenate Strings(w200, "_", w198) -> (w197:string)
                        n131 = String To Path(string=w197) -> (path=w196:path)
                        n132 = call <vilib>:"Check if File or Folder Exists.vi"("path"=w196) -> ("file or folder exists?"=w195:bool, "dup path"=w190:path)  [unwired: 8 in, 1 out]
                        n133 = Not(x=w195) -> (.not. x?=w194:bool)
                      }
                    }
                  }
                  n134 = case shown="True" w173 {
                    tunnel: w171 -> [w210 w212]
                    tunnel: [w210 w211] -> w130
                    frame False {
                    }
                    frame True {
                      n135 = while {
                        tunnel: w212 -> [w214]
                        tunnel: [w213] -> w211
                        i -> [w216]
                        stop <- w217 stop-if-true
                        n136 = Path To String(path=w214) -> (string=w223:string)
                        n137 = Increment(x=w216) -> (x+1=w215:i32)
                        n138 = Number To Decimal String(number=w215) -> (decimal integer string=w221:string)  [unwired: 1 in]
                        n139 = Concatenate Strings(w223, "_", w221) -> (w220:string)
                        n140 = String To Path(string=w220) -> (path=w219:path)
                        n141 = call <vilib>:"Check if File or Folder Exists.vi"("path"=w219) -> ("file or folder exists?"=w218:bool, "dup path"=w213:path)  [unwired: 8 in, 1 out]
                        n142 = Not(x=w218) -> (.not. x?=w217:bool)
                      }
                    }
                  }
                  n143 = call "transfer char run_subvi_13_02_12_JWW.vi"("VISA session"=w185, "Y2 axis settings"=w86, "LKG Path"=w88, "Var1 sweep settings"=w133, "Var2 step settings"=w132, "integration time"=w131, "Input Path"=w130, "Dielectric Constant"=w85, "Sample Properties:"=w129) -> ("Check Cluster"=w126:T20, "Output"=w127:T21, "Graph Cluster"=w125:T22, "error?"=w128:errorcluster)  [unwired: 3 in]
                  n144 = local write "error out"(w128) -> ()
                  n145 = Unbundle By Name(w125) -> ("Linear Sqrt"=w123:cluster{dbl[], "trace":dbl[]}[], "Linear Log"=w122:cluster{dbl[], "trace":dbl[]}[], "Linear Raw"=w111:cluster{dbl[], dbl[]}[], "Saturation Sqrt"=w114:cluster{dbl[], "trace":dbl[]}[], "Saturation Log"=w113:cluster{dbl[], "trace":dbl[]}[], "Saturation Raw"=w110:cluster{dbl[], "trace":dbl[]}[], "Gate Current"=w103:cluster{dbl[], "trace":dbl[]}[])
                  n146 = Index Array(array=w123, index=w121) -> (element=w120:cluster{dbl[], "trace":dbl[]})
                  n147 = Index Array(array=w122, index=w121) -> (element=w119:cluster{dbl[], "trace":dbl[]})
                  n148 = Index Array(array=w114, index=w115) -> (element=w116:cluster{dbl[], "trace":dbl[]})
                  n149 = Index Array(array=w113, index=w115) -> (element=w117:cluster{dbl[], "trace":dbl[]})
                  n150 = Build Array(w120, w119) -> (w118:cluster{dbl[], "trace":dbl[]}[])
                  n151 = Build Array(w116, w117) -> (w112:cluster{dbl[], "trace":dbl[]}[])
                  n152 = Bundle By Name(cluster=w124, "Linear Transfer"=w118, "Linear Raw"=w111, "Saturation Transfer"=w112, "Saturation Raw"=w110, "TRF Gate Current"=w103) -> (w109:T7)
                  n153 = local write "Graph Cluster"(w109) -> ()
                  n154 = local write "Vt Cluster"(w126) -> ()
                  n155 = local write "Char Cluster"(w127) -> ()
                  n156 = property on="Saturation Transfer" class="XYGraph (strict)"("Active Plot"=0, "Plot.YScaleIdx"=0, "Active Plot"=1, "Plot.YScaleIdx"=0) -> ()  [unwired: 2 in, 2 out]
                  n157 = local write "LKG Path"(w88) -> ()
                  n158 = local write "TRF Path"(w130) -> ()
                }
                frame #1 {
                  n159 = local read "Gated SMU4 is..."() -> (w224:bool)
                  n160 = case shown="True" w224 {
                    frame False {
                    }
                    frame True {
                      n161 = local read "Light Bathe Cluster"() -> (w228:T2)
                      n162 = local read "VISA resource name"() -> (w225:refnum<visa-resource-name>)
                      n163 = Unbundle By Name(w228) -> ("TG to BG:"=w227:bool, "TG to BG Durration"=w226:dbl)
                      n164 = case shown="True" w227 {
                        tunnel: w226 -> [_ w230]
                        tunnel: w225 -> [_ w229]
                        frame False {
                        }
                        frame True {
                          n165 = flat-sequence {
                            tunnel: w229 -> [w231]
                            tunnel: w230 -> [w233]
                            tunnel: w229 -> [w234]
                            frame #0 {
                              w232 = u32 1 items=["positive pulse  ", "negative pulse  ", "level high  ", "level low  "] ("trigger signal")
                              n166 = call "HP415xA Op-Trigger Output.vi"("trigger signal"=w232, "VISA session"=w231) -> ()  [unwired: 2 in, 1 out]
                            }
                            frame #1 {
                              n167 = call "Time Delay"("Delay Time (s)"=w233) -> ()  [unwired: 10 in, 1 out]
                            }
                            frame #2 {
                              w235 = u32 0 items=["positive pulse  ", "negative pulse  ", "level high  ", "level low  "] ("trigger signal")
                              n168 = call "HP415xA Op-Trigger Output.vi"("trigger signal"=w235, "VISA session"=w234) -> ()  [unwired: 2 in, 1 out]
                            }
                          }
                        }
                      }
                    }
                  }
                }
                frame #2 {
                  n169 = local read "Gated SMU4 is..."() -> (w236:bool)
                  n170 = case shown="True" w236 {
                    tunnel: w237 -> [_ w300]
                    frame False {
                    }
                    frame True {
                      w276 = 0
                      w282 = 0
                      w326 = "XXX"
                      w329 = "XXX"
                      # "Transfer w/ Gated SMU4"
                      # "This frame takes the measurement settings and sends them to the Transfer subVI for execution (if the \"Transfer\" checkbox is selected on the front panel).\n\nThe data is saved to the folder specified by the user on the front panel with the file name generated by the sample properties.  If the file name already exists, the data is appended to the end of the file.\n\nThe Indicator LED on the front panel should display \"Measuring Transfer\"."
                      n171 = local read "Compliance Cluster"() -> (w305:T6)
                      n172 = local read "TRF Cluster"() -> (w310:T10)
                      n173 = Unbundle By Name(w305) -> ("Var1 sweep settings"=w303:T15, "Var2 step settings"=w304:T16)
                      n174 = local read "TRF Cluster"() -> (w313:T10)
                      n175 = Unbundle By Name(w313) -> ("Start 4"=w312:dbl, "Total Points 2"=w311:u16)
                      n176 = Unbundle By Name(w310) -> ("Start 3"=w309:dbl, "Stop 2"=w308:dbl, "Step 3"=w307:dbl)
                      n177 = local read "TG Dielectric Prop"() -> (w242:T1)
                      n178 = Unbundle By Name(w242) -> ("Dielectric Constant (TG)"=w241:dbl, "Dielectric (d) (TG)"=w238:string)
                      n179 = local read "Gate Current Cluster"() -> (w248:T3)
                      n180 = local read "VISA resource name"() -> (w294:refnum<visa-resource-name>)
                      n181 = Unbundle(w303) -> ("sweep spacing (linear: 0)"=w346:u16, "sweep mode"=w345:bool, "compliance (V)"=w344:dbl, "compliance (A)"=w343:dbl)
                      n182 = Unbundle By Name(w248) -> ("Gate Current (TRF)"=w247:T17)
                      n183 = Unbundle(w304) -> ("compliance (A)"=w342:dbl, "compliance (V)"=w341:dbl)
                      n184 = local read "TRF Cluster"() -> (w295:T10)
                      n185 = Bundle("Start 3"=w309, "Stop 2"=w308, "Step 3"=w307, "sweep spacing (linear: 0)"=w346, "sweep mode"=w345, "compliance (V)"=w344, "compliance (A)"=w343) -> (w293:T18)  [unwired: 1 in]
                      n186 = local read "Sample Properties:"() -> (w244:T9)
                      n187 = local read "TRF Cluster"() -> (w306:T10)
                      n188 = Unbundle By Name(w306) -> ("Integration Time 3"=w291:u32)
                      n189 = Unbundle By Name(w295) -> ("Loop Step"=w298:dbl, "First Step"=w297:dbl)
                      n190 = local read "Saved Folder:"() -> (w263:path)
                      n191 = local write "Status Indicator"(TRUE) -> ()
                      n192 = Multiply(x=w298, y=w300) -> (x*y=w301:dbl)
                      n193 = Unbundle By Name(w244) -> ("Comments"=w246:string)
                      n194 = Add(x=w297, y=w301) -> (x+y=w296:dbl)
                      n195 = Bundle("compliance (A)"=w342, "compliance (V)"=w341, "Start 4"=w312, "Total Points 2"=w311, w296) -> (w292:T19)  [unwired: 1 in]
                      n196 = local read "Saved Folder:"() -> (w269:path)
                      n197 = Bundle By Name(cluster=w295, "Step 4"=w296) -> (w299:T10)
                      n198 = Build Path(base path=w263, name or relative path="TRF_SMU4") -> (appended path=w319:path)
                      n199 = Concatenate Strings(w246, "Gated SMU4" ("string")) -> (w243:string)
                      n200 = local write "TRF Cluster"(w299) -> ()
                      n201 = Build Path(base path=w263, name or relative path="LKG") -> (appended path=w259:path)
                      n202 = Bundle By Name(cluster=w244, "Comments"=w243) -> (w240:T9)
                      n203 = Bundle By Name(cluster=w240, "Dielectric (d)"=w238) -> (w239:T9)
                      n204 = Unbundle(w240) -> ("Index (#)"=w337:string, "Index (ABC)"=w336:string, "Length"=w323:string, "Width"=w325:string, "T (K)"=w302:dbl)  [unwired: 8 out]
                      n205 = Decimal String To Number(string=w323) -> (number=w332:i32)  [unwired: 2 in, 1 out]
                      n206 = Concatenate Strings(w337, w336) -> (w254:string)
                      n207 = Equal?(x=w325, y=w326) -> (x = y?=w327:bool)
                      n208 = Number To Decimal String(number=w332) -> (decimal integer string=w328:string)  [unwired: 1 in]
                      n209 = Equal?(x=w323, y=w329) -> (x = y?=w330:bool)
                      n210 = Build Path(base path=w269, name or relative path="TRF") -> (appended path=w267:path)
                      n211 = Select(t=w329, s=w330, f=w328) -> (s? t:f=w253:string)
                      n212 = call <vilib>:"Check if File or Folder Exists.vi"("path"=w267) -> ("file or folder exists?"=w265:bool, "dup path"=w266:path)  [unwired: 8 in, 1 out]
                      n213 = local read "Graph Cluster"() -> (w285:T7)
                      n214 = property on="Status Indicator" class="Bool (strict)"("BoolText.Text"="Measuring\nTransfer (SMU4)") -> ()  [unwired: 2 in, 2 out]
                      n215 = case shown="False" w265 {
                        tunnel: w266 -> [w365 w366]
                        tunnel: [w364 w366] -> _
                        frame False {
                          n216 = Create Folder(path (use dialog)=w365) -> (created path=w364:path)  [unwired: 2 in, 2 out]
                        }
                        frame True {
                        }
                      }
                      n217 = Decimal String To Number(string=w325) -> (number=w331:i32)  [unwired: 2 in, 1 out]
                      n218 = Number To Decimal String(number=w331) -> (decimal integer string=w324:string)  [unwired: 1 in]
                      n219 = Select(t=w326, s=w327, f=w324) -> (s? t:f=w252:string)
                      n220 = Number To Decimal String(number=w302) -> (decimal integer string=w251:string)  [unwired: 1 in]
                      n221 = call "Build Text3"("T"=w251, "Index"=w254, "Length"=w253, "Width"=w252) -> ("Result"=w255:string)  [unwired: 10 in, 1 out]
                      n222 = call <vilib>:"Check if File or Folder Exists.vi"("path"=w319) -> ("file or folder exists?"=w321:bool, "dup path"=w320:path)  [unwired: 8 in, 1 out]
                      n223 = call <vilib>:"Check if File or Folder Exists.vi"("path"=w259) -> ("file or folder exists?"=w260:bool, "dup path"=w261:path)  [unwired: 8 in, 1 out]
                      n224 = call "Build Text"("T"=w251, "Index"=w254, "Length"=w253, "Width"=w252) -> ("Result"=w340:string)  [unwired: 10 in, 1 out]
                      n225 = case shown="False" w321 {
                        tunnel: w320 -> [w368 w369]
                        tunnel: [w367 w369] -> w318
                        frame False {
                          n226 = Create Folder(path (use dialog)=w368) -> (created path=w367:path)  [unwired: 2 in, 2 out]
                        }
                        frame True {
                        }
                      }
                      n227 = Build Path(base path=w318, name or relative path=w340) -> (appended path=w334:path)
                      n228 = case shown="False" w260 {
                        tunnel: w261 -> [w362 w363]
                        tunnel: [w361 w363] -> w250
                        frame False {
                          n229 = Create Folder(path (use dialog)=w362) -> (created path=w361:path)  [unwired: 2 in, 2 out]
                        }
                        frame True {
                        }
                      }
                      n230 = Build Path(base path=w250, name or relative path=w255) -> (appended path=w258:path)
                      n231 = call <vilib>:"Check if File or Folder Exists.vi"("path"=w334) -> ("file or folder exists?"=w335:bool, "dup path"=w333:path)  [unwired: 8 in, 1 out]
                      n232 = call <vilib>:"Check if File or Folder Exists.vi"("path"=w258) -> ("file or folder exists?"=w257:bool, "dup path"=w256:path)  [unwired: 8 in, 1 out]
                      n233 = case shown="True" w257 {
                        tunnel: w256 -> [w347 w349]
                        tunnel: [w347 w348] -> w249
                        frame False {
                        }
                        frame True {
                          n234 = while {
                            tunnel: w349 -> [w351]
                            tunnel: [w350] -> w348
                            i -> [w353]
                            stop <- w354 stop-if-true
                            n235 = Path To String(path=w351) -> (string=w360:string)
                            n236 = Increment(x=w353) -> (x+1=w352:i32)
                            n237 = Number To Decimal String(number=w352) -> (decimal integer string=w358:string)  [unwired: 1 in]
                            n238 = Concatenate Strings(w360, "_", w358) -> (w357:string)
                            n239 = String To Path(string=w357) -> (path=w356:path)
                            n240 = call <vilib>:"Check if File or Folder Exists.vi"("path"=w356) -> ("file or folder exists?"=w355:bool, "dup path"=w350:path)  [unwired: 8 in, 1 out]
                            n241 = Not(x=w355) -> (.not. x?=w354:bool)
                          }
                        }
                      }
                      n242 = case shown="True" w335 {
                        tunnel: w333 -> [w370 w372]
                        tunnel: [w370 w371] -> w290
                        frame False {
                        }
                        frame True {
                          n243 = while {
                            tunnel: w372 -> [w374]
                            tunnel: [w373] -> w371
                            i -> [w376]
                            stop <- w377 stop-if-true
                            n244 = Path To String(path=w374) -> (string=w383:string)
                            n245 = Increment(x=w376) -> (x+1=w375:i32)
                            n246 = Number To Decimal String(number=w375) -> (decimal integer string=w381:string)  [unwired: 1 in]
                            n247 = Concatenate Strings(w383, "_", w381) -> (w380:string)
                            n248 = String To Path(string=w380) -> (path=w379:path)
                            n249 = call <vilib>:"Check if File or Folder Exists.vi"("path"=w379) -> ("file or folder exists?"=w378:bool, "dup path"=w373:path)  [unwired: 8 in, 1 out]
                            n250 = Not(x=w378) -> (.not. x?=w377:bool)
                          }
                        }
                      }
                      n251 = call "transfer char run_subvi_SMU4_13_02_12_JWW.vi"("VISA session"=w294, "Y2 axis settings"=w247, "LKG Path"=w249, "Var1 sweep settings"=w293, "Var2 step settings"=w292, "integration time"=w291, "Input Path"=w290, "Dielectric Constant"=w241, "Sample Properties:"=w239) -> ("Check Cluster"=w287:T20, "Output"=w288:T21, "Graph Cluster"=w286:T22, "error?"=w289:errorcluster)  [unwired: 3 in]
                      n252 = local write "error out"(w289) -> ()
                      n253 = Unbundle By Name(w286) -> ("Linear Sqrt"=w284:cluster{dbl[], "trace":dbl[]}[], "Linear Log"=w283:cluster{dbl[], "trace":dbl[]}[], "Linear Raw"=w272:cluster{dbl[], dbl[]}[], "Saturation Sqrt"=w275:cluster{dbl[], "trace":dbl[]}[], "Saturation Log"=w274:cluster{dbl[], "trace":dbl[]}[], "Saturation Raw"=w271:cluster{dbl[], "trace":dbl[]}[], "Gate Current"=w264:cluster{dbl[], "trace":dbl[]}[])
                      n254 = Index Array(array=w284, index=w282) -> (element=w281:cluster{dbl[], "trace":dbl[]})
                      n255 = Index Array(array=w283, index=w282) -> (element=w280:cluster{dbl[], "trace":dbl[]})
                      n256 = Index Array(array=w275, index=w276) -> (element=w277:cluster{dbl[], "trace":dbl[]})
                      n257 = Index Array(array=w274, index=w276) -> (element=w278:cluster{dbl[], "trace":dbl[]})
                      n258 = Build Array(w281, w280) -> (w279:cluster{dbl[], "trace":dbl[]}[])
                      n259 = Build Array(w277, w278) -> (w273:cluster{dbl[], "trace":dbl[]}[])
                      n260 = Bundle By Name(cluster=w285, "Linear Transfer"=w279, "Linear Raw"=w272, "Saturation Transfer"=w273, "Saturation Raw"=w271, "TRF Gate Current"=w264) -> (w270:T7)
                      n261 = local write "Graph Cluster"(w270) -> ()
                      n262 = local write "Vt Cluster"(w287) -> ()
                      n263 = local write "Char Cluster"(w288) -> ()
                      n264 = property on="Saturation Transfer" class="XYGraph (strict)"("Active Plot"=0, "Plot.YScaleIdx"=0, "Active Plot"=1, "Plot.YScaleIdx"=0) -> ()  [unwired: 2 in, 2 out]
                      n265 = local write "LKG Path"(w249) -> ()
                      n266 = local write "TRF Path"(w290) -> ()
                    }
                  }
                }
              }
            }
          }
        }
        frame #3 {
          n267 = local write "Status Indicator"(FALSE) -> ()
        }
        frame #4 {
          # "This frame creates the countdown timer for the wait inbetween the\nTransfer and Transport (if both selected)."
          n268 = disable-structure shown="Disabled" {
            frame Disabled {
              n269 = node-c288(1) -> (w398:T12)  [unwired: 1 in]
              n270 = timed-loop {
                timing: w398 -> [_]
                timing-out: [_] -> w397
                i -> [w409]
                stop <- w410 stop-if-true
                n271 = node-c288() -> ()  [unwired: 1 in, 1 out]
                n272 = local read "Wait Cluster"() -> (w402:T5)
                n273 = Unbundle By Name(w402) -> ("Wait Time (s)"=w400:dbl)
                n274 = Multiply(x=w409, y=0.001) -> (x*y=w407:dbl)
                n275 = local read "TRF Cluster"() -> (w403:T10)
                n276 = local read "TSP Cluster"() -> (w404:T11)
                n277 = Unbundle By Name(w404) -> ("Transport"=w405:bool)
                n278 = Unbundle By Name(w403) -> ("Transfer 2"=w406:bool)
                n279 = And(x=w406, y=w405) -> (x .and. y?=w414:bool)
                n280 = Select(t="Waiting...", s=w414, f="Ready") -> (s? t:f=w416:string)
                n281 = property on="Status Indicator" class="Bool (strict)"("BoolText.Text"=w416) -> ()  [unwired: 2 in, 2 out]
                n282 = Select(t=w400, s=w414, f=0) -> (s? t:f=w412:dbl)
                n283 = Subtract(x=w412, y=w407) -> (x-y=w401:dbl)
                n284 = Less Or Equal?(x=w401, y=0) -> (x <= y?=w410:bool)
                n285 = Bundle("Wait Time (s)"=w400, w401) -> (w399:cluster{"Wait Time (s)":dbl, dbl})  [unwired: 1 in]
                n286 = local write "Wait Cluster"(w399) -> ()
                n287 = node-c288() -> ()  [unwired: 1 in, 1 out]
              }
              n288 = node-c288(w397) -> ()  [unwired: 1 out]
            }
            frame Enabled {
            }
          }
          n289 = local read "Light Bathe Cluster"() -> (w385:T2)
          n290 = Unbundle By Name(w385) -> ("TRF to TSP:"=w388:bool, "TRF to TSP Duration"=w387:dbl)
          n291 = local read "VISA resource name"() -> (w386:refnum<visa-resource-name>)
          n292 = case shown="True" w388 {
            tunnel: w387 -> [_ w390]
            tunnel: w386 -> [_ w389]
            frame False {
            }
            frame True {
              n293 = flat-sequence {
                tunnel: w389 -> [w391]
                tunnel: w390 -> [w393]
                tunnel: w389 -> [w394]
                frame #0 {
                  w392 = u32 1 items=["positive pulse  ", "negative pulse  ", "level high  ", "level low  "] ("trigger signal")
                  n294 = call "HP415xA Op-Trigger Output.vi"("trigger signal"=w392, "VISA session"=w391) -> ()  [unwired: 2 in, 1 out]
                }
                frame #1 {
                  n295 = call "Time Delay2"("Delay Time (s)"=w393) -> ()  [unwired: 10 in, 1 out]
                }
                frame #2 {
                  w395 = u32 0 items=["positive pulse  ", "negative pulse  ", "level high  ", "level low  "] ("trigger signal")
                  n296 = call "HP415xA Op-Trigger Output.vi"("trigger signal"=w395, "VISA session"=w394) -> ()  [unwired: 2 in, 1 out]
                }
              }
            }
          }
        }
        frame #5 {
          n297 = local read "TSP Cluster"() -> (w425:T11)
          n298 = Unbundle By Name(w425) -> ("Transport"=w424:bool)
          n299 = case shown="True" w424 {
            frame False {
            }
            frame True {
              n300 = stacked-sequence {
                frame #0 {
                  w458 = "XXX"
                  w462 = "XXX"
                  # "TSP w/o SMU4"
                  # "This frame takes the measurement settings and sends them to the Transport subVI for execution (if the \"Transport\" checkbox is selected on the front panel).\n\nThe data is saved to the folder specified by the user on the front panel with the file name generated by the sample properties.  If the file name already exists, the data is appended to the end of the file.\n\nThe Indicator LED on the front panel should display \"Measuring Transport\"."
                  n301 = local read "Compliance Cluster"() -> (w437:T6)
                  n302 = local read "TSP Cluster"() -> (w449:T11)
                  n303 = local read "Gate Current Cluster"() -> (w427:T3)
                  n304 = Unbundle By Name(w437) -> ("Var1 sweep settings 2"=w436:T15, "Var2 step settings 2"=w435:T16)
                  n305 = local read "TSP Cluster"() -> (w442:T11)
                  n306 = local read "VISA resource name"() -> (w439:refnum<visa-resource-name>)
                  n307 = local read "TSP Cluster"() -> (w440:T11)
                  n308 = Unbundle By Name(w440) -> ("Start"=w445:dbl, "Total Points"=w444:u16, "Step"=w443:dbl)
                  n309 = Unbundle By Name(w449) -> ("Start 2"=w448:dbl, "Stop 3"=w447:dbl, "Step 2"=w446:dbl)
                  n310 = Unbundle By Name(w442) -> ("Integration Time"=w441:u32)
                  n311 = Unbundle By Name(w427) -> ("Gate Current (TSP)"=w426:T17)
                  n312 = Unbundle(w436) -> ("sweep spacing (linear: 0)"=w485:u16, "sweep mode"=w484:bool, "compliance (V)"=w483:dbl, "compliance (A)"=w482:dbl)
                  n313 = Bundle("Start 2"=w448, "Stop 3"=w447, "Step 2"=w446, "sweep spacing (linear: 0)"=w485, "sweep mode"=w484, "compliance (V)"=w483, "compliance (A)"=w482) -> (w481:T23)  [unwired: 1 in]
                  n314 = Unbundle(w435) -> ("compliance (A)"=w480:dbl, "compliance (V)"=w479:dbl)
                  n315 = local read "Saved Folder:"() -> (w438:path)
                  n316 = Bundle("compliance (A)"=w480, "compliance (V)"=w479, "Start"=w445, "Total Points"=w444, "Step"=w443) -> (w478:T24)  [unwired: 1 in]
                  n317 = local read "Sample Properties:"() -> (w474:T9)
                  n318 = local write "Status Indicator"(TRUE) -> ()
                  n319 = Build Path(base path=w438, name or relative path="TSP") -> (appended path=w451:path)
                  n320 = Unbundle(w474) -> ("Index (#)"=w473:string, "Index (ABC)"=w472:string, "Length"=w463:string, "Width"=w459:string, "T (K)"=w433:dbl)  [unwired: 8 out]
                  n321 = Equal?(x=w462, y=w463) -> (x = y?=w464:bool)
                  n322 = property on="Status Indicator" class="Bool (strict)"("BoolText.Text"="Measuring\nTransport") -> ()  [unwired: 2 in, 2 out]
                  n323 = Concatenate Strings(w473, w472) -> (w471:string)
                  n324 = Equal?(x=w458, y=w459) -> (x = y?=w467:bool)
                  n325 = local read "Graph Cluster"() -> (w431:T7)
                  n326 = Decimal String To Number(string=w463) -> (number=w466:i32)  [unwired: 2 in, 1 out]
                  n327 = Decimal String To Number(string=w459) -> (number=w465:i32)  [unwired: 2 in, 1 out]
                  n328 = call <vilib>:"Check if File or Folder Exists.vi"("path"=w451) -> ("file or folder exists?"=w453:bool, "dup path"=w452:path)  [unwired: 8 in, 1 out]
                  n329 = case shown="False" w453 {
                    tunnel: w452 -> [w487 w488]
                    tunnel: [w486 w488] -> w450
                    frame False {
                      n330 = Create Folder(path (use dialog)=w487) -> (created path=w486:path)  [unwired: 2 in, 2 out]
                    }
                    frame True {
                    }
                  }
                  n331 = Number To Decimal String(number=w466) -> (decimal integer string=w461:string)  [unwired: 1 in]
                  n332 = Select(t=w462, s=w464, f=w461) -> (s? t:f=w460:string)
                  n333 = Number To Decimal String(number=w465) -> (decimal integer string=w457:string)  [unwired: 1 in]
                  n334 = Select(t=w458, s=w467, f=w457) -> (s? t:f=w456:string)
                  n335 = call "Build Text2"("T"=w433, "Index"=w471, "Length"=w460, "Width"=w456) -> ("Result"=w455:string)  [unwired: 10 in, 1 out]
                  n336 = Build Path(base path=w450, name or relative path=w455) -> (appended path=w468:path)
                  n337 = call <vilib>:"Check if File or Folder Exists.vi"("path"=w468) -> ("file or folder exists?"=w470:bool, "dup path"=w469:path)  [unwired: 8 in, 1 out]
                  n338 = case shown="True" w470 {
                    tunnel: w469 -> [w489 w491]
                    tunnel: [w489 w490] -> w434
                    frame False {
                    }
                    frame True {
                      n339 = while {
                        tunnel: w491 -> [w493]
                        tunnel: [w492] -> w490
                        i -> [w495]
                        stop <- w496 stop-if-true
                        n340 = Path To String(path=w493) -> (string=w502:string)
                        n341 = Increment(x=w495) -> (x+1=w494:i32)
                        n342 = Number To Decimal String(number=w494) -> (decimal integer string=w500:string)  [unwired: 1 in]
                        n343 = Concatenate Strings(w502, "_", w500) -> (w499:string)
                        n344 = String To Path(string=w499) -> (path=w498:path)
                        n345 = call <vilib>:"Check if File or Folder Exists.vi"("path"=w498) -> ("file or folder exists?"=w497:bool, "dup path"=w492:path)  [unwired: 8 in, 1 out]
                        n346 = Not(x=w497) -> (.not. x?=w496:bool)
                      }
                    }
                  }
                  n347 = call "transport char run_subvi_2013_09_11_JWa.vi"("VISA session"=w439, "Y2 axis settings"=w426, "Var1 sweep settings"=w481, "Var2 step settings"=w478, "integration time"=w441, "Path"=w434, "Sample Properties:"=w474) -> ("Graph Cluster"=w432:T25, "error?"=w477:errorcluster)  [unwired: 6 in, 1 out]
                  n348 = local write "error out"(w477) -> ()
                  n349 = Unbundle By Name(w432) -> ("Transport"=w429:cluster{dbl[], dbl[]}[], "Gate Current"=w428:cluster{dbl[], dbl[]}[])
                  n350 = local write "TSP Path"(w434) -> ()
                  n351 = Bundle By Name(cluster=w431, "Transport"=w429, "TSP Gate Current"=w428) -> (w430:T7)
                  n352 = local write "Graph Cluster"(w430) -> ()
                }
                frame #1 {
                  n353 = local read "Gated SMU4 is..."() -> (w503:bool)
                  n354 = case shown="True" w503 {
                    frame False {
                    }
                    frame True {
                      n355 = local read "Light Bathe Cluster"() -> (w507:T2)
                      n356 = local read "VISA resource name"() -> (w504:refnum<visa-resource-name>)
                      n357 = Unbundle By Name(w507) -> ("TG to BG (TSP):"=w506:bool, "TG to BG Durration 3"=w505:dbl)
                      n358 = case shown="True" w506 {
                        tunnel: w505 -> [_ w509]
                        tunnel: w504 -> [_ w508]
                        frame False {
                        }
                        frame True {
                          n359 = flat-sequence {
                            tunnel: w508 -> [w510]
                            tunnel: w509 -> [w512]
                            tunnel: w508 -> [w513]
                            frame #0 {
                              w511 = u32 1 items=["positive pulse  ", "negative pulse  ", "level high  ", "level low  "] ("trigger signal")
                              n360 = call "HP415xA Op-Trigger Output.vi"("trigger signal"=w511, "VISA session"=w510) -> ()  [unwired: 2 in, 1 out]
                            }
                            frame #1 {
                              n361 = call "Time Delay3"("Delay Time (s)"=w512) -> ()  [unwired: 10 in, 1 out]
                            }
                            frame #2 {
                              w514 = u32 0 items=["positive pulse  ", "negative pulse  ", "level high  ", "level low  "] ("trigger signal")
                              n362 = call "HP415xA Op-Trigger Output.vi"("trigger signal"=w514, "VISA session"=w513) -> ()  [unwired: 2 in, 1 out]
                            }
                          }
                        }
                      }
                    }
                  }
                }
                frame #2 {
                  # "TSP w/ SMU4"
                  n363 = local read "Gated SMU4 is..."() -> (w515:bool)
                  n364 = case shown="True" w515 {
                    frame False {
                    }
                    frame True {
                      w548 = "XXX"
                      w552 = "XXX"
                      # "This frame takes the measurement settings and sends them to the Transport subVI for execution (if the \"Transport\" checkbox is selected on the front panel).\n\nThe data is saved to the folder specified by the user on the front panel with the file name generated by the sample properties.  If the file name already exists, the data is appended to the end of the file.\n\nThe Indicator LED on the front panel should display \"Measuring Transport\"."
                      n365 = local read "Compliance Cluster"() -> (w527:T6)
                      n366 = local read "TSP Cluster"() -> (w539:T11)
                      n367 = local read "Gate Current Cluster"() -> (w517:T3)
                      n368 = Unbundle By Name(w527) -> ("Var1 sweep settings 2"=w526:T15, "Var2 step settings 2"=w525:T16)
                      n369 = local read "TSP Cluster"() -> (w532:T11)
                      n370 = local read "VISA resource name"() -> (w529:refnum<visa-resource-name>)
                      n371 = local read "TSP Cluster"() -> (w530:T11)
                      n372 = Unbundle By Name(w530) -> ("Start"=w535:dbl, "Total Points"=w534:u16, "Step"=w533:dbl)
                      n373 = Unbundle By Name(w539) -> ("Start 2"=w538:dbl, "Stop 3"=w537:dbl, "Step 2"=w536:dbl)
                      n374 = Unbundle By Name(w532) -> ("Integration Time"=w531:u32)
                      n375 = Unbundle By Name(w517) -> ("Gate Current (TSP)"=w516:T17)
                      n376 = Unbundle(w526) -> ("sweep spacing (linear: 0)"=w575:u16, "sweep mode"=w574:bool, "compliance (V)"=w573:dbl, "compliance (A)"=w572:dbl)
                      n377 = Bundle("Start 2"=w538, "Stop 3"=w537, "Step 2"=w536, "sweep spacing (linear: 0)"=w575, "sweep mode"=w574, "compliance (V)"=w573, "compliance (A)"=w572) -> (w571:T23)  [unwired: 1 in]
                      n378 = Unbundle(w525) -> ("compliance (A)"=w570:dbl, "compliance (V)"=w569:dbl)
                      n379 = local read "Saved Folder:"() -> (w528:path)
                      n380 = Bundle("compliance (A)"=w570, "compliance (V)"=w569, "Start"=w535, "Total Points"=w534, "Step"=w533) -> (w568:T24)  [unwired: 1 in]
                      n381 = local read "Sample Properties:"() -> (w564:T9)
                      n382 = local write "Status Indicator"(TRUE) -> ()
                      n383 = Build Path(base path=w528, name or relative path="TSP_SMU4") -> (appended path=w541:path)
                      n384 = Unbundle(w564) -> ("Index (#)"=w563:string, "Index (ABC)"=w562:string, "Length"=w553:string, "Width"=w549:string, "T (K)"=w523:dbl)  [unwired: 8 out]
                      n385 = Equal?(x=w552, y=w553) -> (x = y?=w554:bool)
                      n386 = property on="Status Indicator" class="Bool (strict)"("BoolText.Text"="     Measuring\nTransport SMU4") -> ()  [unwired: 2 in, 2 out]
                      n387 = Concatenate Strings(w563, w562) -> (w561:string)
                      n388 = Equal?(x=w548, y=w549) -> (x = y?=w557:bool)
                      n389 = local read "Graph Cluster"() -> (w521:T7)
                      n390 = Decimal String To Number(string=w553) -> (number=w556:i32)  [unwired: 2 in, 1 out]
                      n391 = Decimal String To Number(string=w549) -> (number=w555:i32)  [unwired: 2 in, 1 out]
                      n392 = call <vilib>:"Check if File or Folder Exists.vi"("path"=w541) -> ("file or folder exists?"=w543:bool, "dup path"=w542:path)  [unwired: 8 in, 1 out]
                      n393 = case shown="False" w543 {
                        tunnel: w542 -> [w577 w578]
                        tunnel: [w576 w578] -> w540
                        frame False {
                          n394 = Create Folder(path (use dialog)=w577) -> (created path=w576:path)  [unwired: 2 in, 2 out]
                        }
                        frame True {
                        }
                      }
                      n395 = Number To Decimal String(number=w556) -> (decimal integer string=w551:string)  [unwired: 1 in]
                      n396 = Select(t=w552, s=w554, f=w551) -> (s? t:f=w550:string)
                      n397 = Number To Decimal String(number=w555) -> (decimal integer string=w547:string)  [unwired: 1 in]
                      n398 = Select(t=w548, s=w557, f=w547) -> (s? t:f=w546:string)
                      n399 = call "Build Text6"("T"=w523, "Index"=w561, "Length"=w550, "Width"=w546) -> ("Result"=w545:string)  [unwired: 10 in, 1 out]
                      n400 = Build Path(base path=w540, name or relative path=w545) -> (appended path=w558:path)
                      n401 = call <vilib>:"Check if File or Folder Exists.vi"("path"=w558) -> ("file or folder exists?"=w560:bool, "dup path"=w559:path)  [unwired: 8 in, 1 out]
                      n402 = case shown="True" w560 {
                        tunnel: w559 -> [w579 w581]
                        tunnel: [w579 w580] -> w524
                        frame False {
                        }
                        frame True {
                          n403 = while {
                            tunnel: w581 -> [w583]
                            tunnel: [w582] -> w580
                            i -> [w585]
                            stop <- w586 stop-if-true
                            n404 = Path To String(path=w583) -> (string=w592:string)
                            n405 = Increment(x=w585) -> (x+1=w584:i32)
                            n406 = Number To Decimal String(number=w584) -> (decimal integer string=w590:string)  [unwired: 1 in]
                            n407 = Concatenate Strings(w592, "_", w590) -> (w589:string)
                            n408 = String To Path(string=w589) -> (path=w588:path)
                            n409 = call <vilib>:"Check if File or Folder Exists.vi"("path"=w588) -> ("file or folder exists?"=w587:bool, "dup path"=w582:path)  [unwired: 8 in, 1 out]
                            n410 = Not(x=w587) -> (.not. x?=w586:bool)
                          }
                        }
                      }
                      n411 = call "transport char run_subvi_2014_02_18_SMU4_JWa.vi"("VISA session"=w529, "Y2 axis settings"=w516, "Var1 sweep settings"=w571, "Var2 step settings"=w568, "integration time"=w531, "Path"=w524, "Sample Properties:"=w564) -> ("Graph Cluster"=w522:T25, "error?"=w567:errorcluster)  [unwired: 6 in, 1 out]
                      n412 = local write "error out"(w567) -> ()
                      n413 = Unbundle By Name(w522) -> ("Transport"=w519:cluster{dbl[], dbl[]}[], "Gate Current"=w518:cluster{dbl[], dbl[]}[])
                      n414 = local write "TSP Path"(w524) -> ()
                      n415 = Bundle By Name(cluster=w521, "Transport"=w519, "TSP Gate Current"=w518) -> (w520:T7)
                      n416 = local write "Graph Cluster"(w520) -> ()
                    }
                  }
                }
              }
            }
          }
        }
        frame #6 {
          n417 = local write "Status Indicator"(FALSE) -> ()
          n418 = property on="Status Indicator" class="Bool (strict)"("BoolText.Text"="Ready") -> ()  [unwired: 2 in, 2 out]
        }
        frame #7 {
          n419 = disable-structure shown="Disabled" {
            disable-tunnel: w596 -> [w598 _]
            disable-tunnel: w595 -> [w597 _]
            frame Disabled {
              n420 = node-c288(100) -> (w603:T12)  [unwired: 3 in]
              n421 = timed-loop {
                timing: w603 -> [_]
                timing-out: [_] -> w602
                tunnel: w598 -> [w614]
                tunnel: w597 -> [w613]
                tunnel: ["Stop \nCountdown"] -> _
                i -> [w619]
                stop <- w609 stop-if-true
                n422 = node-c288() -> ()  [unwired: 1 in, 1 out]
                n423 = local read "TRF Cluster"() -> (w608:T10)
                n424 = Unbundle By Name(w608) -> ("Loop Wait"=w606:dbl)
                n425 = Multiply(x=0.1, y=w619) -> (x*y=w617:dbl)
                n426 = Equal?(x=w613, y=w614) -> (x = y?=w615:bool)
                n427 = Select(t=0, s=w615, f=w606) -> (s? t:f=w611:dbl)
                n428 = Subtract(x=w611, y=w617) -> (x-y=w605:dbl)
                n429 = Less Or Equal To 0?(x=w605) -> (x <= 0?=w610:bool)
                n430 = Or(x=w610, y="Stop \nCountdown") -> (x .or. y?=w609:bool)
                n431 = Bundle("Loop Wait"=w606, w605) -> (w607:cluster{"Loop Wait":dbl, dbl})  [unwired: 1 in]
                n432 = property on="Status Indicator" class="Bool (strict)"("BoolText.Text"="Waiting...") -> ()  [unwired: 2 in, 2 out]
                n433 = local write "Wait Cluster"(w607) -> ()
                n434 = node-c288() -> ()  [unwired: 1 in, 1 out]
              }
              n435 = node-c288(w602) -> (w599:errorcluster)
              n436 = property on="Status Indicator" class="Bool (strict)"(error in=w599, "BoolText.Text"="Ready") -> ()  [unwired: 1 in, 2 out]
            }
            frame Enabled {
            }
          }
        }
      }
      n437 = local write "VISA resource name out"(w9) -> ()
    }
  }
